vi "Hardware-EPTxDataCalPoints.vi"(8 "Loading":bool, 9 "Max CAD":sgl, 10 "EPTxData":T1) -> ()   [LabVIEW 2016, in "DSI-RT.lvlib"]
uses:
  DSI-RT.lvlib
  <vilib>/Powertrain Controls/Device Drivers/Engine Position Tracking/EPTx/RevA/RT/Controls/EPTxData.ctl
  <vilib>/addons/Software Calibration Management/xSCM/CalPoint.xnode
  <vilib>/addons/Software Calibration Management/xSCM/ni_scm.dll
  <vilib>/Powertrain Controls/Device Drivers/Engine Position Tracking/EPTx/RevA/RT/EPTx - RevA - RT.lvlib
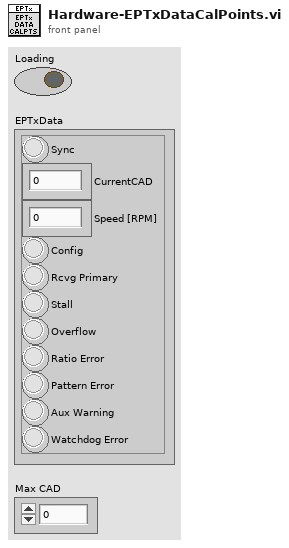
[diagram p1: front panel]
types:
  T1 = typedef "EPTx - RevA - RT.lvlib/EPTxData.ctl" = cluster{"Sync":bool, "CurrentCAD":sgl, "Speed [RPM]":sgl, "Config":bool, "Rcvg Primary":bool, "Stall":bool, "Overflow":bool, "Ratio Error":bool, "Pattern Error":bool, "Aux Warning":bool, "Watchdog Error":bool}
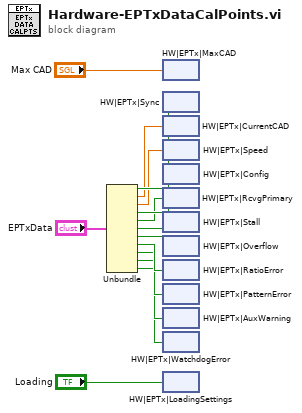
[diagram p0: block diagram]
diagram:
  n1 = Unbundle("EPTxData") -> ("Sync"=w12:bool, "CurrentCAD"=w11:sgl, "Speed [RPM]"=w10:sgl, "Config"=w9:bool, "Rcvg Primary"=w8:bool, "Stall"=w2:bool, "Overflow"=w1:bool, "Ratio Error"=w7:bool, "Pattern Error"=w6:bool, "Aux Warning"=w5:bool, "Watchdog Error"=w4:bool)
  n2 = xnode "HW|EPTx|MaxCAD"("Value"="Max CAD") -> ()
  n3 = xnode "HW|EPTx|Sync"("Value"=w12) -> ()
  n4 = xnode "HW|EPTx|CurrentCAD"("Value"=w11) -> ()
  n5 = xnode "HW|EPTx|Speed"("Value"=w10) -> ()
  n6 = xnode "HW|EPTx|Config"("Value"=w9) -> ()
  n7 = xnode "HW|EPTx|RcvgPrimary"("Value"=w8) -> ()
  n8 = xnode "HW|EPTx|Stall"("Value"=w2) -> ()
  n9 = xnode "HW|EPTx|Overflow"("Value"=w1) -> ()
  n10 = xnode "HW|EPTx|RatioError"("Value"=w7) -> ()
  n11 = xnode "HW|EPTx|PatternError"("Value"=w6) -> ()
  n12 = xnode "HW|EPTx|AuxWarning"("Value"=w5) -> ()
  n13 = xnode "HW|EPTx|WatchdogError"("Value"=w4) -> ()
  n14 = xnode "HW|EPTx|LoadingSettings"("Value"="Loading") -> ()
